vi "SequenceMotion.vi"(8 "error in (no error)":errorcluster, 10 "sub-systems in":refnum<class "sub-systems.lvclass">, 11 "VXMMotionManager in":refnum<class "VXMMotionManager.lvclass">) -> (0 "error out":errorcluster, 1 "Motions Finished = T":bool, 2 "sub-systems out":refnum<class "sub-systems.lvclass">, 3 "VXMMotionManager out":refnum<class "VXMMotionManager.lvclass">, 4 "Axis Number":i32, 5 "Position":T1)   [LabVIEW 2019, in "VXMMotionManager.lvclass"]
doc: "This VI contains logic and VXM Motion Controller commands. (It does probably too much.)\nIt is designed to be called in a loop, check the DEMO VI in the class library.\nThis VI starts motion on one axis, then polls the motion until it ends, and then starts motion on the next axis. When motion on all four axes is complete:\n Motion Finished indicator = T\n IF move was extablish Home, THEN Set Homing Complete bit and send UI message\n IF move was a Position move, THEN Send ACK to APAR sequencer"
uses:
  VXMMotionManager.lvclass
  sub-systems/sub-systems.lvclass
  MoveAllAbsoluteStates.ctl
  APARMainSubvis/VXM Public API/singleAxisMoveDef.ctl
  APARMainSubvis/VXM Public API/mmWaveAxis.ctl
  VXMMotionManager.lvclass/VXMMotionManager.ctl
  Support/MessageAPI/UIMessage.ctl
  MotionTypes.ctl
  SendMessage/SendMessage.lvclass
  VSMx2/VXMx2.lvclass
panel:
  out "State":T3
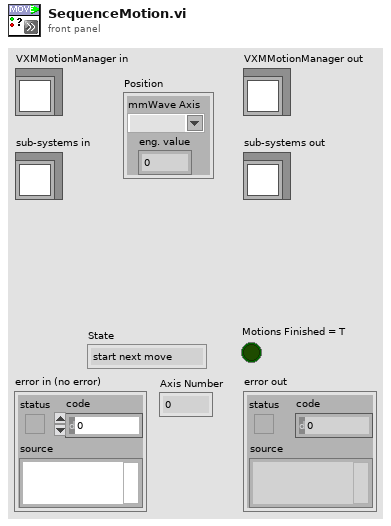
[diagram p1: front panel]
types:
  T1 = typedef "singleAxisMoveDef.ctl" = cluster{"mmWave Axis":T2, "eng. value":dbl}
  T2 = typedef "mmWaveAxis.ctl" = string
  T3 = typedef "VXMMotionManager.lvclass/MoveAllAbsoluteStates.ctl" = enum16{"start next move", "wait motion end"}
  T4 = typedef "UIMessage.ctl" = cluster{"EventCode":i32, "Numeric":dbl, "String":string, "Variant":variant}
  T5 = typedef "MotionTypes.ctl" = enum16{"Homing", "AllAbsolute", "AllHome", "Position", "OneAxisHome", "Clear"}
  T6 = typedef "Velmex VXM.lvlib/VXM Axis.ctl" = u16
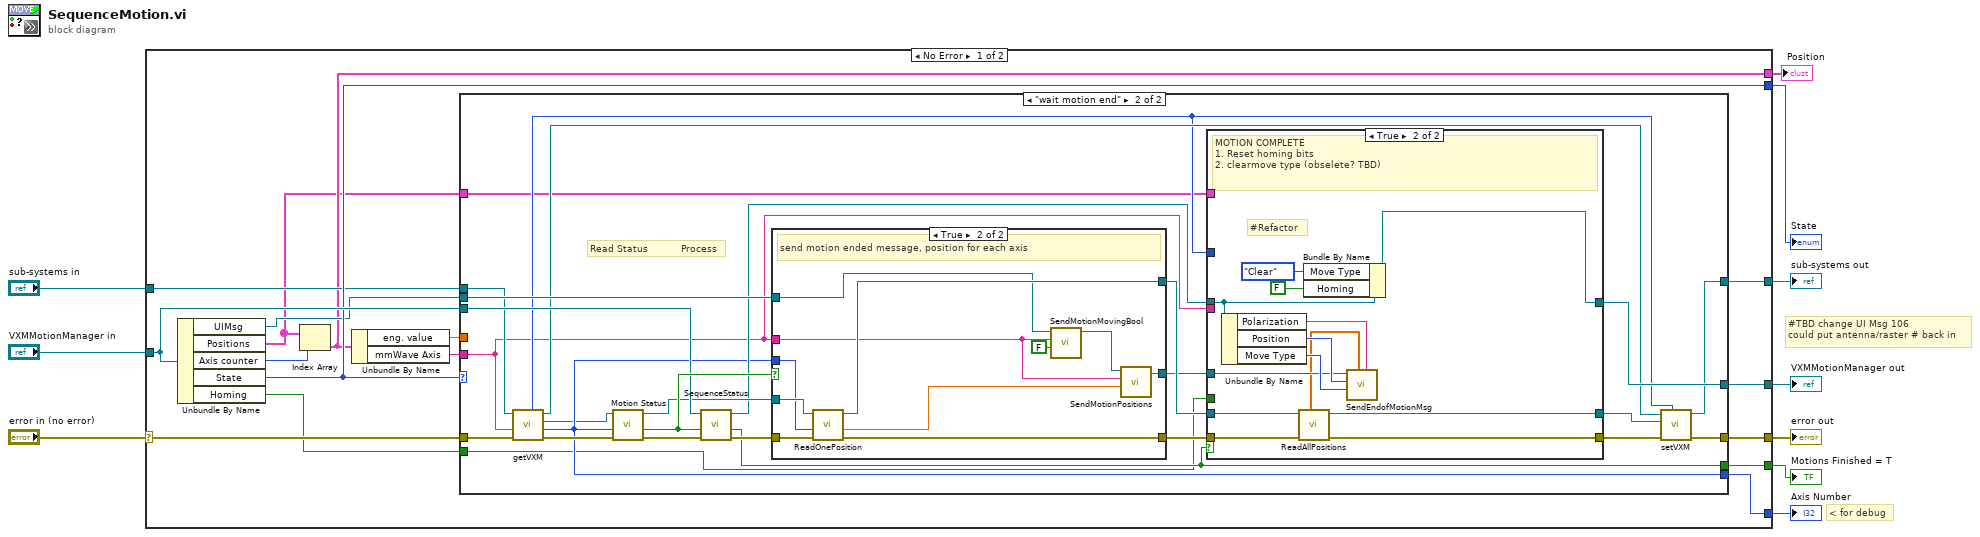
[diagram p0: block diagram]
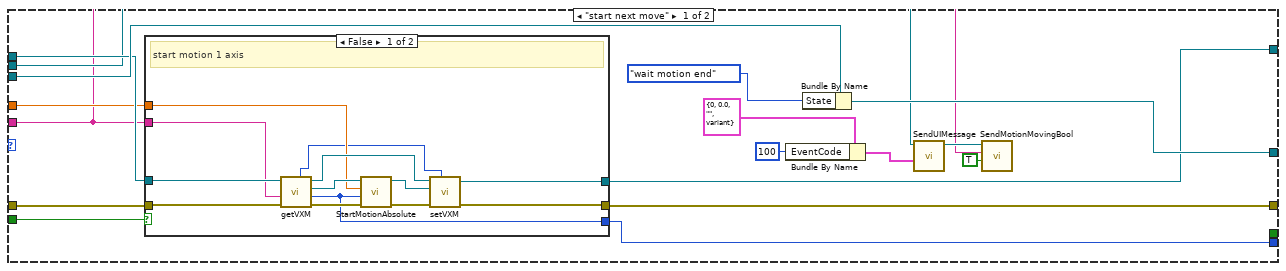
[diagram p2: hidden frame]
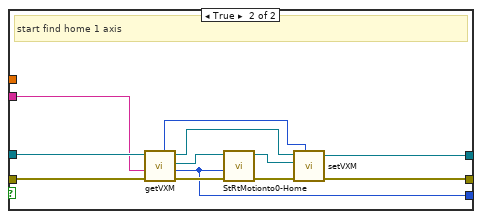
[diagram p3: hidden frame]
diagram:
  # "#TBD change UI Msg 106\ncould put antenna/raster # back in"
  # "< for debug"
  n1 = case shown="No Error" "error in (no error)" {
    selector: "error in (no error)" -> [w25 w127]
    tunnel: [w24 w127] -> w10
    tunnel: [w23 w126] -> w9
    tunnel: "VXMMotionManager in" -> [w26 w126]
    tunnel: [w22 _] -> w4
    tunnel: [w17 _] -> w3
    tunnel: [w21 _] -> w2
    tunnel: "sub-systems in" -> [w20 w125]
    tunnel: [w19 w125] -> w5
    tunnel: [w14 _] -> w1
    frame No Error {
      n2 = Unbundle By Name(w26) -> ("UIMsg"=w18:refnum<class "SendMessage.lvclass">, "Positions"=w11:T1[], "Axis counter"=w12:i32, "State"=w21:T3, "Homing"=w13:bool)
      n3 = Index Array(array=w11, index=w12) -> (element=w17:T1)
      n4 = Unbundle By Name(w17) -> ("eng. value"=w16:dbl, "mmWave Axis"=w15:T2)
      n5 = case shown="\"wait motion end\"" w21 {
        tunnel: w26 -> [w43 w91]
        tunnel: [w42 w85] -> w23
        tunnel: w25 -> [w41 w81]
        tunnel: [w40 w76] -> w24
        tunnel: [_ w88] -> w22
        tunnel: w18 -> [w32 w93]
        tunnel: w20 -> [w35 w79]
        tunnel: [w34 w73] -> w19
        tunnel: w13 -> [w33 w72]
        tunnel: w16 -> [w31 _]
        tunnel: w15 -> [w28 w70]
        tunnel: [w30 w80] -> w14
        tunnel: w11 -> [_ w69]
        frame "start next move" {
          n6 = case shown="False" w33 {
            tunnel: w41 -> [w53 w66]
            tunnel: [w48 w64] -> w40
            tunnel: w35 -> [w55 w67]
            tunnel: [w49 w65] -> w34
            tunnel: w31 -> [w47 _]
            tunnel: w28 -> [w46 w61]
            tunnel: [w45 w60] -> w30
            frame False {
              # "start motion 1 axis"
              n7 = call "getVXM.vi"("error in (no error)"=w53, "mmWave Axis Name"=w46, "sub-systems in"=w55) -> ("error out"=w54:errorcluster, "Axis (1..4)"=w45:T6, "VXMx2 out"=w51:refnum<class "VXMx2.lvclass">, "sub-systems out"=w56:refnum<class "sub-systems.lvclass">, "Sub-syst number"=w44:i32)  [unwired: 4 in]
              n8 = call "StartMotionAbsolute.vi"("error in (no error)"=w54, "Axis (1..4)"=w45, "Absolute Position, mm or deg."=w47, "VXMx2 in"=w51) -> ("error out"=w52:errorcluster, "VXMx2 out"=w50:refnum<class "VXMx2.lvclass">)  [unwired: 6 in]
              n9 = call "setVXM.vi"("Sub-syst number"=w44, "error in (no error)"=w52, "VXMn"=w50, "sub-systems in"=w56) -> ("error out"=w48:errorcluster, "sub-systems out"=w49:refnum<class "sub-systems.lvclass">)  [unwired: 6 in]
            }
            frame True {
              # "start find home 1 axis"
              n10 = call "getVXM.vi"("error in (no error)"=w66, "mmWave Axis Name"=w61, "sub-systems in"=w67) -> ("error out"=w63:errorcluster, "Axis (1..4)"=w60:T6, "VXMx2 out"=w58:refnum<class "VXMx2.lvclass">, "sub-systems out"=w68:refnum<class "sub-systems.lvclass">, "Sub-syst number"=w57:i32)  [unwired: 4 in]
              n11 = call "StRtMotionto0-Home.vi"("error in (no error)"=w63, "Axis (1..4)"=w60, "VXMx2 in"=w58) -> ("error out"=w62:errorcluster, "VXMx2 out"=w59:refnum<class "VXMx2.lvclass">)  [unwired: 7 in]
              n12 = call "setVXM.vi"("Sub-syst number"=w57, "error in (no error)"=w62, "VXMn"=w59, "sub-systems in"=w68) -> ("error out"=w64:errorcluster, "sub-systems out"=w65:refnum<class "sub-systems.lvclass">)  [unwired: 6 in]
            }
          }
          n13 = Bundle By Name(cluster=T4 {"EventCode"=0, "Numeric"=0.0, "String"="", "Variant"=variant} ("UIMsg"), "EventCode"=100) -> (w37:T4)
          n14 = Bundle By Name(cluster=w43, "State"=MoveAllAbsoluteStates."wait motion end") -> (w42:refnum<class "VXMMotionManager.lvclass">)
          n15 = call-dynamic "SendUIMessage.vi"("UIMsg"=w37, "SendMessage in"=w32) -> ("SendMessage out"=w29:refnum<class "SendMessage.lvclass">)  [unwired: 8 in, 1 out]
          n16 = call "SendMotionMovingBool.vi"("Axis True= Moving"=TRUE, "mmWave Axis Name"=w28, "SendMessage in"=w29) -> ()  [unwired: 7 in, 2 out]
        }
        frame "wait motion end" {
          # "Read Status           Process"
          n17 = call "getVXM.vi"("error in (no error)"=w81, "mmWave Axis Name"=w70, "sub-systems in"=w79) -> ("error out"=w82:errorcluster, "Axis (1..4)"=w80:T6, "VXMx2 out"=w78:refnum<class "VXMx2.lvclass">, "sub-systems out"=w75:refnum<class "sub-systems.lvclass">, "Sub-syst number"=w71:i32)  [unwired: 4 in]
          n18 = call "Motion Status.vi"("error in (no error)"=w82, "Axis (1..4)"=w80, "VXMx2 in"=w78) -> ("error out"=w94:errorcluster, "Motion Stopped"=w92:bool, "VXMx2 out"=w89:refnum<class "VXMx2.lvclass">)  [unwired: 5 in, 1 out]
          n19 = call "SequenceStatus.vi"("error in (no error)"=w94, "Motion Stopped"=w92, "VXMMotionManager in"=w91) -> ("error out"=w90:errorcluster, "last axis = True"=w88:bool, "VXMMotionManager out"=w86:refnum<class "VXMMotionManager.lvclass">)  [unwired: 6 in]
          n20 = case shown="True" w92 {
            tunnel: w93 -> [w111 w118]
            tunnel: w80 -> [_ w121]
            tunnel: w90 -> [w112 w124]
            tunnel: w89 -> [w113 w123]
            tunnel: [w112 w122] -> w87
            tunnel: [w113 w120] -> w84
            tunnel: [w111 w117] -> w83
            tunnel: w70 -> [_ w114]
            frame False {
              # "still moving"
            }
            frame True {
              # "send motion ended message, position for each axis"
              n21 = call "ReadOnePosition.vi"("error in (no error)"=w124, "Axis (1..4)"=w121, "VXMx2 in"=w123) -> ("error out"=w122:errorcluster, "Position, eng units"=w115:dbl, "VXMx2 out"=w120:refnum<class "VXMx2.lvclass">)  [unwired: 6 in]
              n22 = call "SendMotionMovingBool.vi"("Axis True= Moving"=FALSE, "mmWave Axis Name"=w114, "SendMessage in"=w118) -> ("SendMessage out"=w116:refnum<class "SendMessage.lvclass">)  [unwired: 7 in, 1 out]
              n23 = call "SendMotionPositions.vi"("Axis Position, eng."=w115, "mmWave Axis Name"=w114, "SendMessage in"=w116) -> ("SendMessage out"=w117:refnum<class "SendMessage.lvclass">)  [unwired: 7 in, 1 out]
            }
          }
          n24 = case shown="True" w88 {
            tunnel: w87 -> [w96 w101]
            tunnel: [w96 w106] -> w77
            tunnel: [w97 w98] -> w85
            tunnel: w86 -> [w97 w108]
            tunnel: w84 -> [w95 w100]
            tunnel: [w95 w107] -> w74
            tunnel: w83 -> [_ w103]
            tunnel: w72 -> [_ _]
            tunnel: w71 -> [_ _]
            tunnel: w70 -> [_ _]
            tunnel: w69 -> [_ _]
            frame False {
            }
            frame True {
              # "#Refactor"
              # "MOTION COMPLETE\n1. Reset homing bits\n2. clearmove type (obselete? TBD)"
              n25 = Unbundle By Name(w108) -> ("Polarization"=w102:string, "Position"=w104:i32, "Move Type"=w105:T5)
              n26 = call "ReadAllPositions.vi"("error in (no error)"=w101, "VXMx2 in"=w100) -> ("error out"=w106:errorcluster, "VXMx2 out"=w107:refnum<class "VXMx2.lvclass">, "All Positions, eng units"=w99:dbl[])  [unwired: 2 in, 5 out]
              n27 = Bundle By Name(cluster=w108, "Move Type"=MotionTypes."Clear", "Homing"=FALSE) -> (w98:refnum<class "VXMMotionManager.lvclass">)
              n28 = call "SendEndofMotionMsg.vi"("Polarization"=w102, "All Positions, eng units"=w99, "Move Type"=w105, "Position"=w104, "SendMessage in"=w103) -> ()  [unwired: 5 in, 2 out]
            }
          }
          n29 = call "setVXM.vi"("Sub-syst number"=w71, "error in (no error)"=w77, "VXMn"=w74, "sub-systems in"=w75) -> ("error out"=w76:errorcluster, "sub-systems out"=w73:refnum<class "sub-systems.lvclass">)  [unwired: 6 in]
        }
      }
    }
    frame Error {
    }
  }
  "error out" <- w10
  "VXMMotionManager out" <- w9
  "sub-systems out" <- w5
  "Motions Finished = T" <- w4
  "State" <- w2
  "Axis Number" <- w1
  "Position" <- w3
